vi "Build Previous Version Project.vi"(8 "Error In":errorcluster) -> ()   [LabVIEW 2017]
uses:
  <vilib>/AppBuilder/AB_API_Simple/Build (path).vi
  <vilib>/AppBuilder/AB_API_Simple/NI_App_Builder_API.lvlib
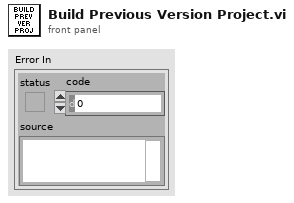
[diagram p1: front panel]
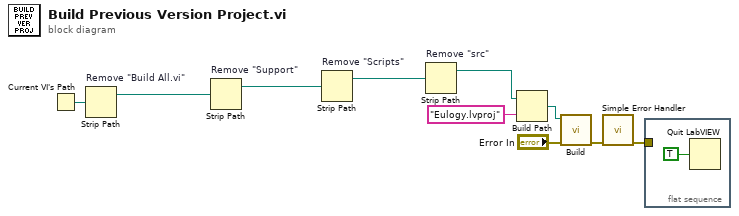
[diagram p0: block diagram]
diagram:
  n1 = Current VI's Path() -> (path=w4:path)
  n2 = Strip Path "Remove \"Build All.vi\""(path=w4) -> (stripped path=w2:path)  [unwired: 1 out]
  n3 = Strip Path "Remove \"Support\""(path=w2) -> (stripped path=w1:path)  [unwired: 1 out]
  n4 = Strip Path "Remove \"Scripts\""(path=w1) -> (stripped path=w8:path)  [unwired: 1 out]
  n5 = Strip Path "Remove \"src\""(path=w8) -> (stripped path=w7:path)  [unwired: 1 out]
  n6 = Build Path(base path=w7, name or relative path="Eulogy.lvproj") -> (appended path=w5:path)
  n7 = call-poly <vilib>:"Build.vi"("error in (no error)"="Error In", "Path to project"=w5) -> ("error out"=w9:errorcluster)  [unwired: 8 in, 1 out]
  n8 = call <vilib>:"Simple Error Handler.vi"("error in (no error)"=w9) -> ("error out"=w3:errorcluster)  [unwired: 4 in, 4 out]
  n9 = flat-sequence {
    tunnel: w3 -> [_]
    frame #0 {
      n10 = Quit LabVIEW(quit? (T)=TRUE) -> ()
    }
  }
